vi "1.vi"(9 "Range end":dbl=10.0, 10 "Step":dbl=1.0, 11 "Range start":dbl) -> (3 "Array":string[](array[string]))   [LabVIEW 2020]
uses:
  044b8177-aabe-489d-8260-c17b0245c5cb.vi
  <vilib>/Comparison/Less/Less Functor/Less Functor.lvclass
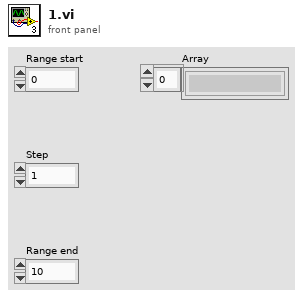
[diagram p1: front panel]
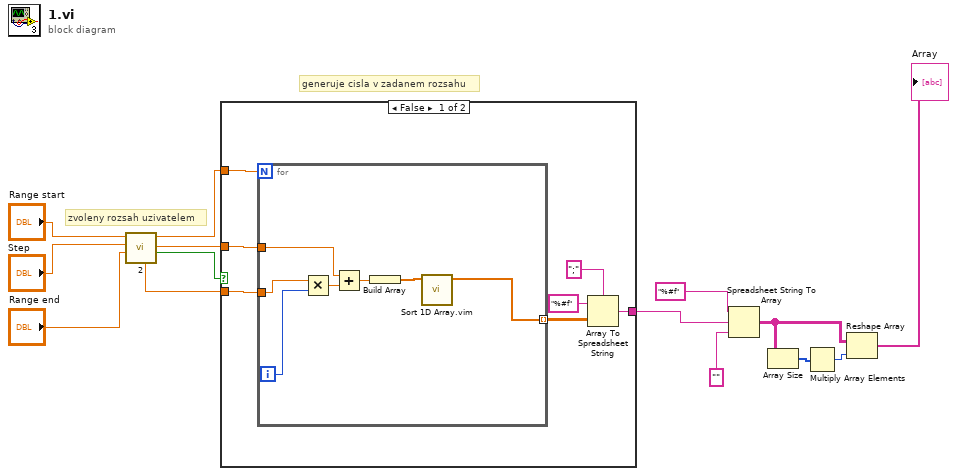
[diagram p0: block diagram]
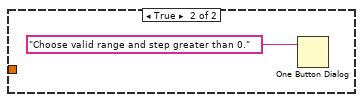
[diagram p2: hidden frame]
diagram:
  # "generuje cisla v zadanem rozsahu"
  # "zvoleny rozsah uzivatelem"
  n1 = call "2.vi"("Range end"="Range end", "Step in"="Step", "Range start in"="Range start") -> ("Boolean"=w3:bool, "Range start out"=w4:dbl, "Numeric"=w1:dbl, "Step out"=w2:dbl)  [unwired: 5 in]
  n2 = case shown="False" w3 {
    tunnel: w2 -> [w21 _]
    tunnel: w4 -> [w20 _]
    tunnel: w1 -> [w19 _]
    tunnel: [w15 _] -> w11
    frame False {
      n3 = for {
        N: w19 -> [_]
        tunnel: w20 -> [w25]
        tunnel: w21 -> [w27]
        tunnel: [w22] -> w16 mode=indexing
        i -> [w28]
        n4 = Multiply(x=w27, y=w28) -> (x*y=w26:dbl)
        n5 = Add(x=w25, y=w26) -> (x+y=w24:dbl)
        n6 = Build Array(w24) -> (w23:dbl[])
        n7 = call "Sort 1D Array.vim"("unsorted array"=w23) -> ("sorted array"=w22:dbl[])  [unwired: 10 in]
      }
      n8 = Array To Spreadsheet String(delimiter (Tab)=";", array=w16, 3:"%#f" ("format string")) -> (spreadsheet string=w15:string)
    }
    frame True {
      n9 = One Button Dialog(message="Choose valid range and step greater than 0.") -> ()  [unwired: 1 in, 1 out]
    }
  }
  n10 = Spreadsheet String To Array(format string="%#f", spreadsheet string=w11, array type (2D Dbl)="") -> (array=w9:string[][])  [unwired: 1 in]
  n11 = Array Size(array=w9) -> (size(s)=w8:i32[])
  n12 = Multiply Array Elements(1:w8) -> (0:w7:i32)
  n13 = Reshape Array(w9, w7) -> (→"Array":string[])
